vi "Day 3 Task 2.vi"() -> ()   [LabVIEW 2018]
panel:
  out "life support rating":u32
  out "CO2":u32
  out "CO2 scrubber rating: keep":bool
  out "oxygen":u32
  out "oxygen gen rating: keep":bool
  out "gamma rate":i32[](array[numeric])
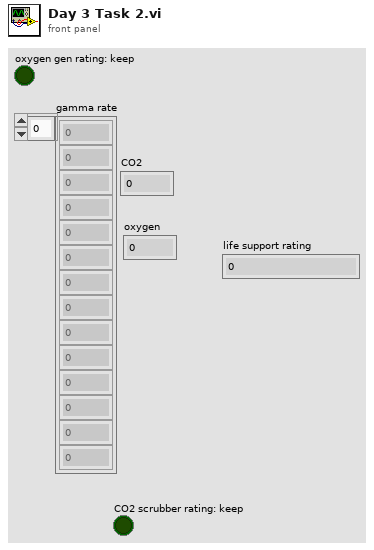
[diagram p1: front panel]
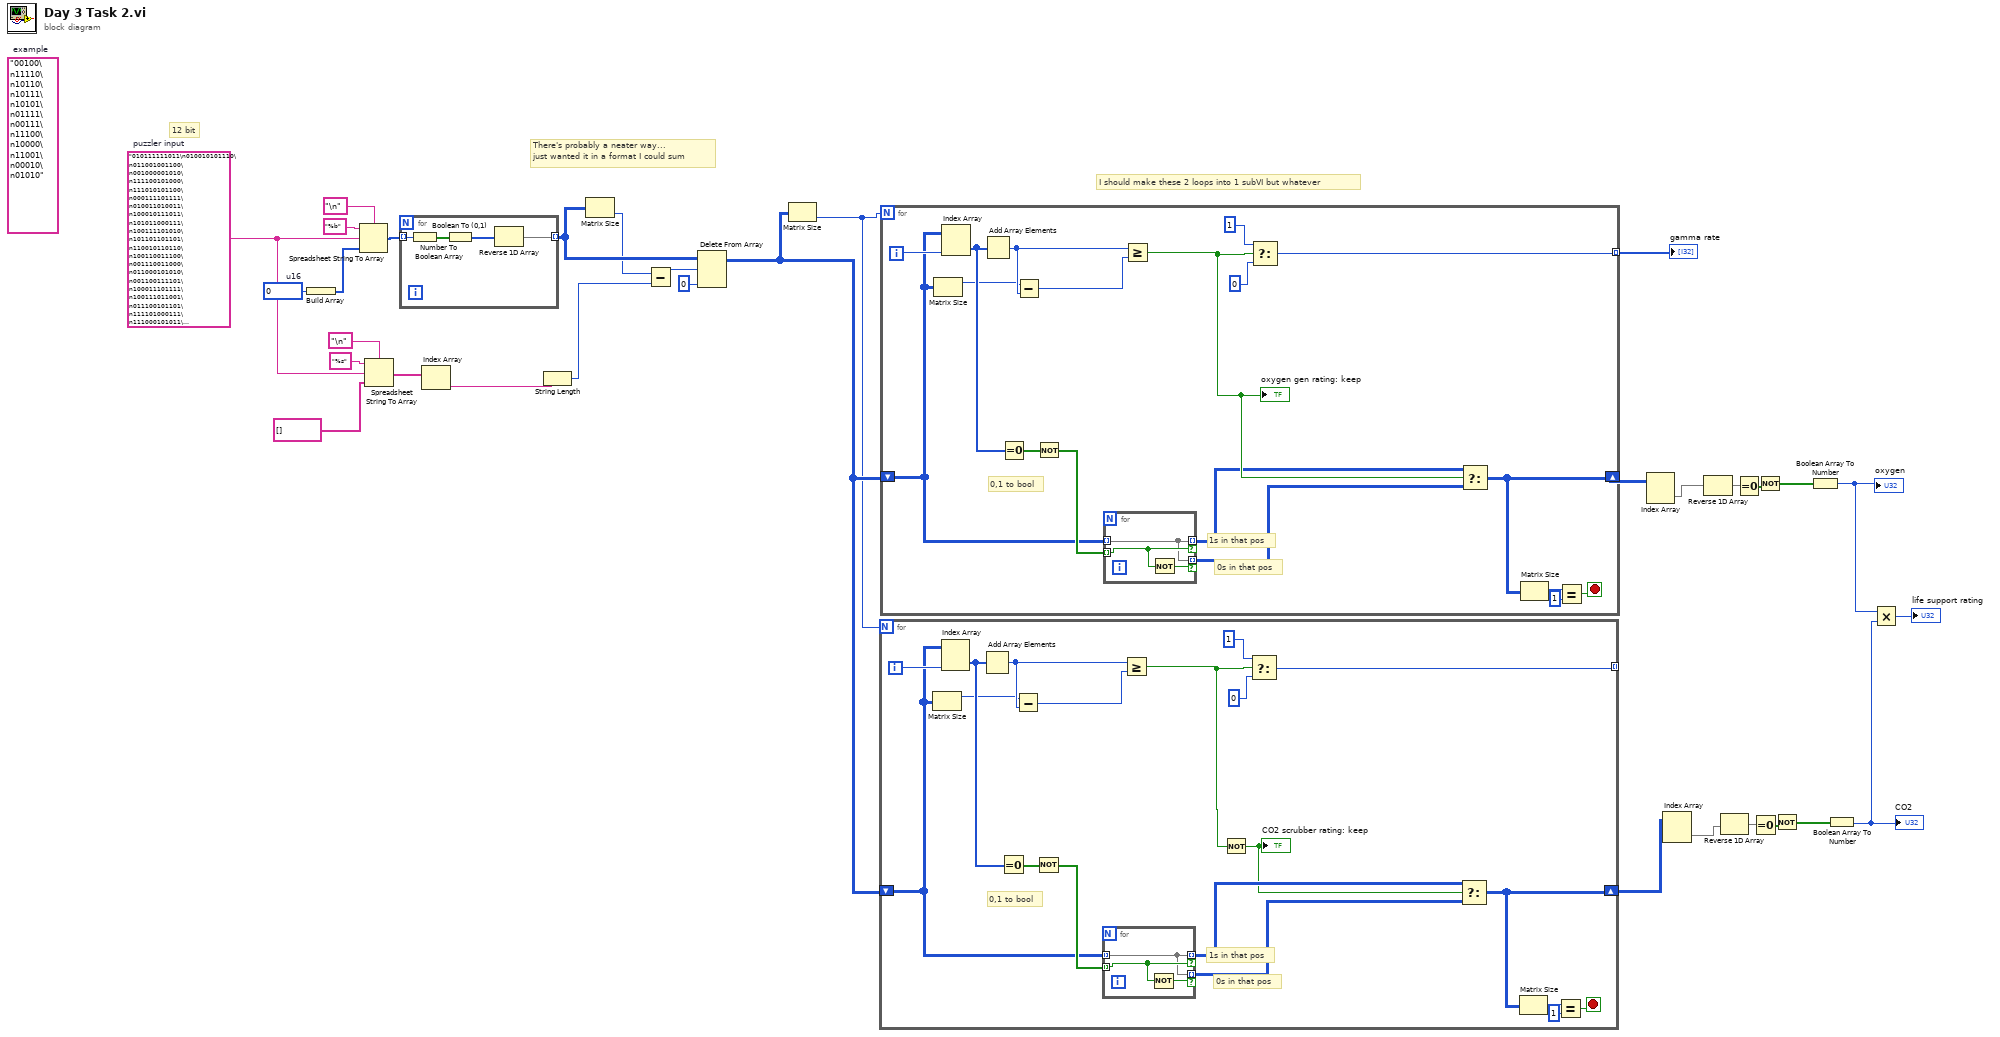
[diagram p0: block diagram]
diagram:
  w1 = "010111111011\n010010101110\n011001001100\n001000001010\n111100101000\n111010101100\n000111101111\n010011010011\n100010111011\n101011000111\n100111101010\n101101101101\n110010110110\n100110011100\n001110011000\n011000101010\n001100111101\n100011101111\n100111011001\n011100101101\n111101000111\n111000101011\n001001000101\n010110011000\n110100100001\n010010010011\n100100100100\n011011001000\n111101011101\n101011110011\n110011101101\n001001000100\n100111101110\n101101101010\n111110101000\n111011011001\n111110101101\n110101010100\n011100110000\n000010111110\n111011111111\n010111111110\n101001110101\n001111010100\n001111110001\n000010000000\n01..."  # puzzler input
  w30 = u16 0  # u16
  (unwired) "00100\n11110\n10110\n10111\n10101\n01111\n00111\n11100\n10000\n11001\n00010\n01010"  # example
  # "I should make these 2 loops into 1 subVI but whatever"
  # "12 bit"
  # "There's probably a neater way...\njust wanted it in a format I could sum"
  n1 = Build Array(w30) -> (w26:u16[])
  n2 = Spreadsheet String To Array(delimiter (Tab)="\n", format string="%b", spreadsheet string=w1, array type (2D Dbl)=w26) -> (array=w29:u16[])
  n3 = Spreadsheet String To Array(delimiter (Tab)="\n", format string="%s", spreadsheet string=w1, array type (2D Dbl)=string[] []) -> (array=w21:string[])
  n4 = for {
    tunnel: w29 -> [w36] mode=indexing
    tunnel: [w34] -> w28 mode=indexing
    n5 = Number To Boolean Array(number=w36) -> (Boolean array=w35:bool[])
    n6 = Boolean To (0,1)(Boolean=w35) -> (0, 1=w33:i16[])
    n7 = Reverse 1D Array(array=w33) -> (reversed array=w34:i16[])
  }
  n8 = Index Array(array=w21) -> (element=w20:string)  [unwired: 1 in]
  n9 = String Length(string=w20) -> (length=w18:i32)
  n10 = Matrix Size(0:w28) -> (2:w27:i32)  [unwired: 1 out]
  n11 = Subtract(x=w27, y=w18) -> (x-y=w19:i32)
  n12 = Delete From Array(array=w28, length=w19, index (col)=0 ("disabled index (col)")) -> (array with subset deleted=w11:i16[][])  [unwired: 1 in, 1 out]
  n13 = Matrix Size(0:w11) -> (2:w10:i32)  [unwired: 1 out]
  n14 = for {
    N: w10 -> [_]
    tunnel: [w54] -> _ mode=indexing
    shift-right: [w41] -> w6
    shift-left: w11 -> [w43]
    i -> [w55]
    stop <- w38 stop-if-true
    # "0s in that pos"
    # "1s in that pos"
    # "0,1 to bool"
    n15 = Matrix Size(0:w43) -> (1:w42:i32)  [unwired: 1 out]
    n16 = Index Array(array=w43, index (col)=w55) -> (element=w49:i16[])  [unwired: 1 in]
    n17 = Add Array Elements(numeric array=w49) -> (sum=w50:i16)
    n18 = Equal To 0?(x=w49) -> (x = 0?=w48:bool[])
    n19 = Subtract(x=w42, y=w50) -> (x-y=w51:i32)
    n20 = Not(x=w48) -> (.not. x?=w46:bool[])
    n21 = for {
      tunnel: w43 -> [w57] mode=indexing
      tunnel: w46 -> [w58] mode=indexing
      tunnel: [w57] -> w45 mode=indexing if=w58
      tunnel: [w57] -> w44 mode=indexing if=w56
      n22 = Not(x=w58) -> (.not. x?=w56:bool)
    }
    n23 = Greater Or Equal?(x=w50, y=w51) -> (x >= y?=w47:bool)
    n24 = Not(x=w47) -> (.not. x?=w37:bool)
    "CO2 scrubber rating: keep" <- w37
    n25 = Select(t=1, s=w47, f=0 ("x-y")) -> (s? t:f=w54:i32)
    n26 = Select(t=w45, s=w37, f=w44) -> (s? t:f=w41:i16[][])
    n27 = Matrix Size(0:w41) -> (1:w40:i32)  [unwired: 1 out]
    n28 = Equal?(x=w40, y=1) -> (x = y?=w38:bool)
  }
  n29 = for {
    N: w10 -> [_]
    tunnel: [w75] -> w25 mode=indexing
    shift-right: [w62] -> w16
    shift-left: w11 -> [w64]
    i -> [w76]
    stop <- w59 stop-if-true
    # "0s in that pos"
    # "1s in that pos"
    # "0,1 to bool"
    n30 = Matrix Size(0:w64) -> (1:w63:i32)  [unwired: 1 out]
    n31 = Index Array(array=w64, index (col)=w76) -> (element=w70:i16[])  [unwired: 1 in]
    n32 = Add Array Elements(numeric array=w70) -> (sum=w71:i16)
    n33 = Equal To 0?(x=w70) -> (x = 0?=w69:bool[])
    n34 = Subtract(x=w63, y=w71) -> (x-y=w72:i32)
    n35 = Not(x=w69) -> (.not. x?=w67:bool[])
    n36 = for {
      tunnel: w64 -> [w78] mode=indexing
      tunnel: w67 -> [w79] mode=indexing
      tunnel: [w78] -> w66 mode=indexing if=w79
      tunnel: [w78] -> w65 mode=indexing if=w77
      n37 = Not(x=w79) -> (.not. x?=w77:bool)
    }
    n38 = Greater Or Equal?(x=w71, y=w72) -> (x >= y?=w68:bool)
    "oxygen gen rating: keep" <- w68
    n39 = Select(t=1, s=w68, f=0 ("x-y")) -> (s? t:f=w75:i32)
    n40 = Select(t=w66, s=w68, f=w65) -> (s? t:f=w62:i16[][])
    n41 = Matrix Size(0:w62) -> (1:w61:i32)  [unwired: 1 out]
    n42 = Equal?(x=w61, y=1) -> (x = y?=w59:bool)
  }
  "gamma rate" <- w25
  n43 = Index Array(array=w16) -> (element=w15:i16[])  [unwired: 2 in]
  n44 = Index Array(array=w6) -> (element=w5:i16[])  [unwired: 2 in]
  n45 = Reverse 1D Array(array=w15) -> (reversed array=w14:i16[])
  n46 = Reverse 1D Array(array=w5) -> (reversed array=w7:i16[])
  n47 = Equal To 0?(x=w14) -> (x = 0?=w13:bool[])
  n48 = Equal To 0?(x=w7) -> (x = 0?=w8:bool[])
  n49 = Not(x=w13) -> (.not. x?=w12:bool[])
  n50 = Not(x=w8) -> (.not. x?=w9:bool[])
  n51 = Boolean Array To Number(Boolean array=w12) -> (number=w4:u32)
  "oxygen" <- w4
  n52 = Boolean Array To Number(Boolean array=w9) -> (number=w3:u32)
  "CO2" <- w3
  n53 = Multiply(x=w4, y=w3) -> (x*y=→"life support rating":u32)
